vi "CLC_Switch_TRxMode_0188.vi"(8 "error in (no error)":errorcluster, 10 "Text Ring":u16(ring)=1 items=["Standby", "TX", "RX"], 11 "TCPIPin":T1={"address"="192.168.100.111", "remote port or service name"=5025, "timeout ms (60000)"=10000}) -> (0 "error out":errorcluster, 1 "OK?":bool, 3 "TCPIPin 2":T1={"address"="192.168.100.111", "remote port or service name"=5025, "timeout ms (60000)"=10000})   [LabVIEW 2023]
panel:
  out "data out":string
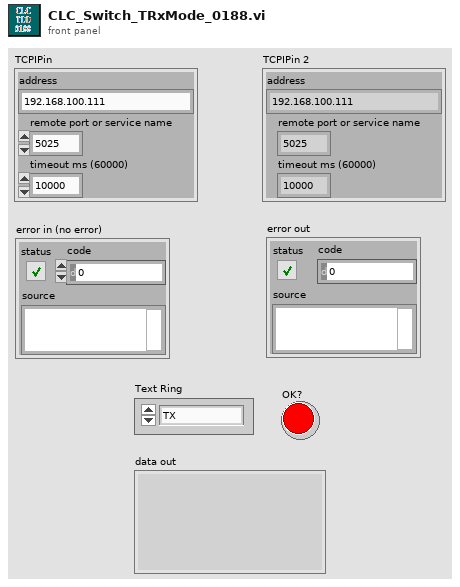
[diagram p1: front panel]
types:
  T1 = cluster{"address":string, "remote port or service name":u16, "timeout ms (60000)":i32}
  T2 = enum16{"Standard", "Buffered", "CRLF", "Immediate"}
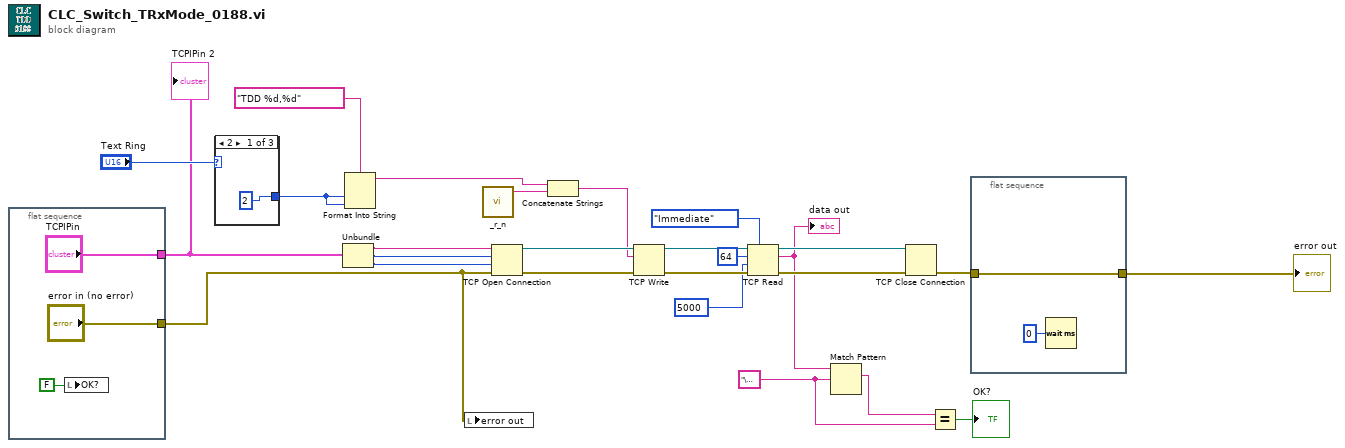
[diagram p0: block diagram]
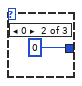
[diagram p2: hidden frame]
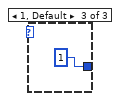
[diagram p3: hidden frame]
diagram:
  w6 = "\u0000" ("string")
  n1 = flat-sequence {
    tunnel: ["TCPIPin"] -> w25
    tunnel: ["error in (no error)"] -> w24
    frame #0 {
      n2 = local write "OK?"(FALSE ("OK?")) -> ()
    }
  }
  n3 = case shown="2" "Text Ring" {
    tunnel: [2 0 1] -> w1
    frame 2 {
    }
    frame 0 {
    }
    frame 1, Default {
    }
  }
  n4 = Unbundle(w25) -> ("address"=w20:string, "remote port or service name"=w19:u16, "timeout ms (60000)"=w18:i32)
  n5 = Format Into String(format string="TDD %d,%d" ("data in"), w1, w1) -> (resulting string=w16:string)  [unwired: 2 in, 1 out]
  n6 = local write "error out"(w24) -> ()
  n7 = call "_r_n.vi"() -> ("command"=w2:string)  [unwired: 5 in]
  n8 = TCP Open Connection(address=w20, remote port or service name=w19, timeout ms (60000)=w18, error in (no error)=w24) -> (connection ID=w23:refnum<k5>, error out=w22:errorcluster)  [unwired: 1 in]
  n9 = Concatenate Strings(w16, w2) -> (w21:string)
  n10 = TCP Write(connection ID=w23, data in=w21, error in (no error)=w22) -> (connection ID out=w14:refnum<k5>, error out=w15:errorcluster)  [unwired: 1 in, 1 out]
  n11 = TCP Read(connection ID=w14, bytes to read=64, error in (no error)=w15, 7:T2."Immediate" ("mode (standard)"), 9:5000 ("timeout ms (25000)")) -> (connection ID out=w13:refnum<k5>, data out=w8:string, error out=w12:errorcluster)
  "data out" <- w8
  n12 = Match Pattern(string=w8, regular expression=w6) -> (match substring=w7:string)  [unwired: 1 in, 3 out]
  n13 = TCP Close Connection(connection ID=w13, error in (no error)=w12) -> (error out=w4:errorcluster)  [unwired: 1 in, 1 out]
  n14 = Equal?(x=w7, y=w6) -> (x = y?=→"OK?":bool)
  n15 = flat-sequence {
    tunnel: w4 -> [w34]
    tunnel: [w34] -> w3
    frame #0 {
      n16 = Wait (ms)(milliseconds to wait=u32 0) -> ()  [unwired: 1 out]
    }
  }
  "error out" <- w3
  "TCPIPin 2" <- w25
